vi "COP Logger.vi"() -> ()   [LabVIEW 2009]
panel:
  in  "stop":bool
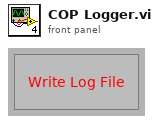
[diagram p1: front panel]
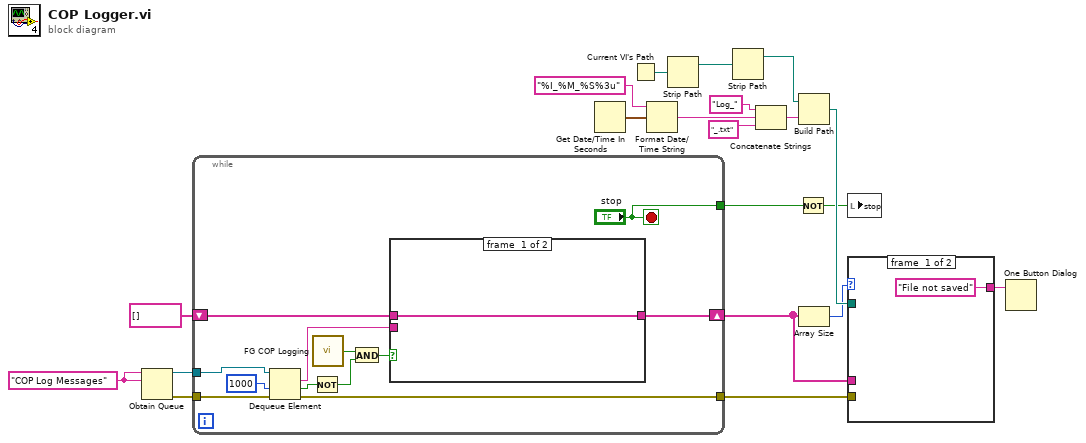
[diagram p0: block diagram]
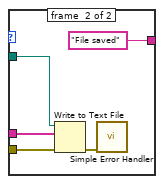
[diagram p2: hidden frame]
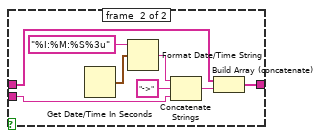
[diagram p3: hidden frame]
diagram:
  w18 = "COP Log Messages" ("name (unnamed)")
  n1 = Obtain Queue(name (unnamed)=w18, element data type=w18) -> (queue out=w20:refnum<queue>, error out=w19:errorcluster)  [unwired: 3 in, 1 out]
  n2 = while {
    tunnel: w20 -> [w32]
    tunnel: w19 -> [w31]
    shift-right: [w27] -> w8
    shift-left: string[] [] -> [w28]
    tunnel: [w26] -> w16
    tunnel: ["stop"] -> w4
    stop <- "stop" stop-if-true
    n3 = Dequeue Element(queue=w32, timeout in ms (-1)=1000, error in (no error)=w31) -> (element=w29:string, timed out?=w25:bool, error out=w26:errorcluster)  [unwired: 1 out]
    n4 = Not(x=w25) -> (.not. x?=w21:bool)
    n5 = call "FG COP Logging.vi"() -> ("Logging? out"=w22:bool)  [unwired: 2 in]
    n6 = And(x=w22, y=w21) -> (x .and. y?=w23:bool)
    n7 = case shown="True" w23 {
      tunnel: w29 -> [_ w35]
      tunnel: w28 -> [w33 w41]
      tunnel: [w33 w40] -> w27
      frame #0 {
      }
      frame #1 {
        n8 = Get Date/Time In Seconds() -> (seconds since 1Jan1904=w39:timestamp)
        n9 = Format Date/Time String(time format string (%c)="%I:%M:%S%3u", seconds (now)=w39) -> (date/time string=w36:string)  [unwired: 1 in]
        n10 = Concatenate Strings(w36, "->" ("string"), w35) -> (w37:string)
        n11 = Build Array (concatenate)(w41, w37) -> (w40:string[])
      }
    }
  }
  n12 = Get Date/Time In Seconds() -> (seconds since 1Jan1904=w11:timestamp)
  n13 = Current VI's Path() -> (path=w13:path)
  n14 = Format Date/Time String(time format string (%c)="%I_%M_%S%3u", seconds (now)=w11) -> (date/time string=w10:string)  [unwired: 1 in]
  n15 = Strip Path(path=w13) -> (stripped path=w2:path)  [unwired: 1 out]
  n16 = Strip Path(path=w2) -> (stripped path=w1:path)  [unwired: 1 out]
  n17 = Concatenate Strings("Log_" ("name or relative path"), w10, "_.txt" ("string")) -> (w15:string)
  n18 = Not(x=w4) -> (.not. x?=w3:bool)
  n19 = Build Path(base path=w1, name or relative path=w15) -> (appended path=w12:path)
  n20 = Array Size(array=w8) -> (size(s)=w7:i32)
  n21 = local write "stop"(w3) -> ()
  n22 = case shown="0" w7 {
    tunnel: w8 -> [_ w47]
    tunnel: w16 -> [_ w46]
    tunnel: w12 -> [_ w45]
    tunnel: ["File not saved" ("message") "File saved" ("message")] -> w5
    frame #0 {
    }
    frame #1 {
      n23 = Write to Text File(file (use dialog)=w45, text=w47, error in=w46) -> (error out=w44:errorcluster)  [unwired: 1 in, 2 out]
      n24 = call <vilib>:"Simple Error Handler.vi"("error in (no error)"=w44) -> ()  [unwired: 4 in, 5 out]
    }
  }
  n25 = One Button Dialog(message=w5) -> ()  [unwired: 1 in, 1 out]
